vi "Create.vi"(8 "error in (no error)":errorcluster, 10 "Response":refnum<class "Response.lvclass">, 11 "Request":refnum<class "Request.lvclass">) -> (0 "error out":errorcluster, 3 "API Message out":refnum<class "API Message.lvclass">)   [LabVIEW 2023, in "API Message.lvclass"]
uses:
  API Message.lvclass
  Request/Request.lvclass
  Response/Response.lvclass
  API Message.lvclass/API Message.ctl
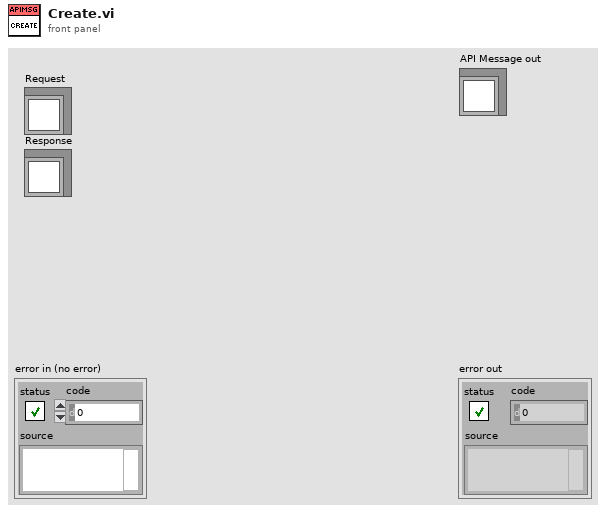
[diagram p1: front panel]
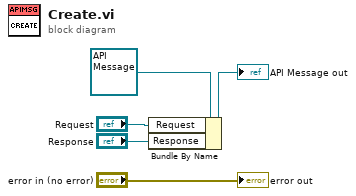
[diagram p0: block diagram]
diagram:
  n1 = Bundle By Name(cluster=refnum<class "API Message.lvclass"> refnum ("API Message in"), "Request"="Request", "Response"="Response") -> (→"API Message out":refnum<class "API Message.lvclass">)
  "error out" <- "error in (no error)"
